vi "Get Client Operation.vi"(8 "error in (no error)":errorcluster, 11 "Client Message in":refnum<class "Client Message.lvclass">) -> (0 "error out":errorcluster, 2 "Client Operation":T1, 3 "Client Message out":refnum<class "Client Message.lvclass">)   [LabVIEW 2020, in "obs-websocket.lvlib" / "Client Message.lvclass"]
uses:
  Client Message.lvclass
  Client Operation.ctl
  Client Message.lvclass/Client Message.ctl
  obs-websocket.lvlib
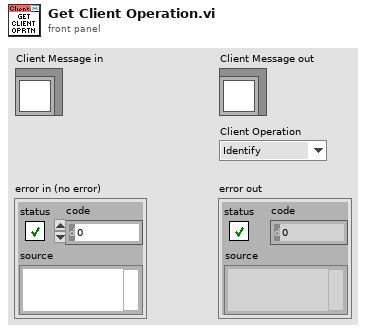
[diagram p1: front panel]
types:
  T1 = typedef "obs-websocket.lvlib/Client Operation.ctl" = enum16{"Identify", "Reidentify", "Request", "RequestBatch"}
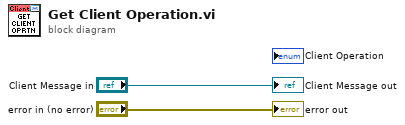
[diagram p0: block diagram]
diagram:
  "error out" <- "error in (no error)"
  "Client Message out" <- "Client Message in"
